vi "DmFET_Underway_Graphed.vi"() -> ()   [LabVIEW 2022 SP3]
uses:
  <vilib>/Utility/file.llb/Write Delimited Spreadsheet (string).vi
panel:
  out "TC_Controller":dbl
  out "BiasBatt- V":dbl
  out "BiasBatt+ V":dbl
  out "MainBatt V":dbl
  out "Ib":dbl
  out "Ik":dbl
  out "Vk_std":dbl
  out "Vk":dbl
  out "Vrse_std":dbl
  out "Vrse":dbl
  out "Vrse_std vs Time":waveform(dbl)(graph)
  out "Vrse vs Time":waveform(dbl)(graph)
  out "Loop #":i32
  in  "milliseconds to wait":u32=2000
  in  "stop":bool
  in  "file (use dialog)":path
  in  "DURA1 COM":refnum<visa-resource-name>="COM24"
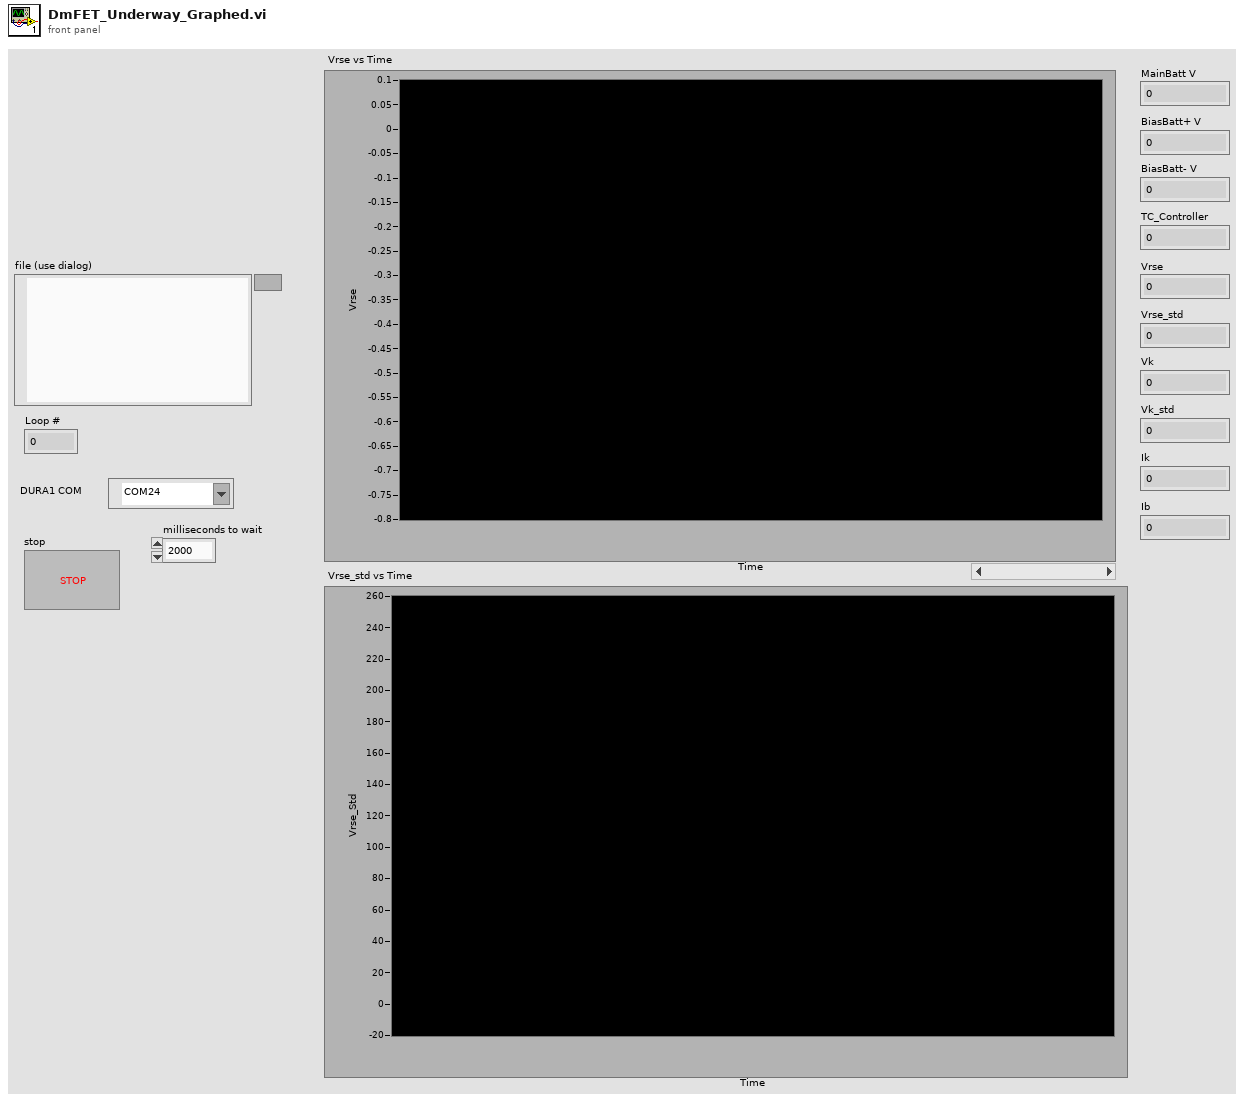
[diagram p1: front panel]
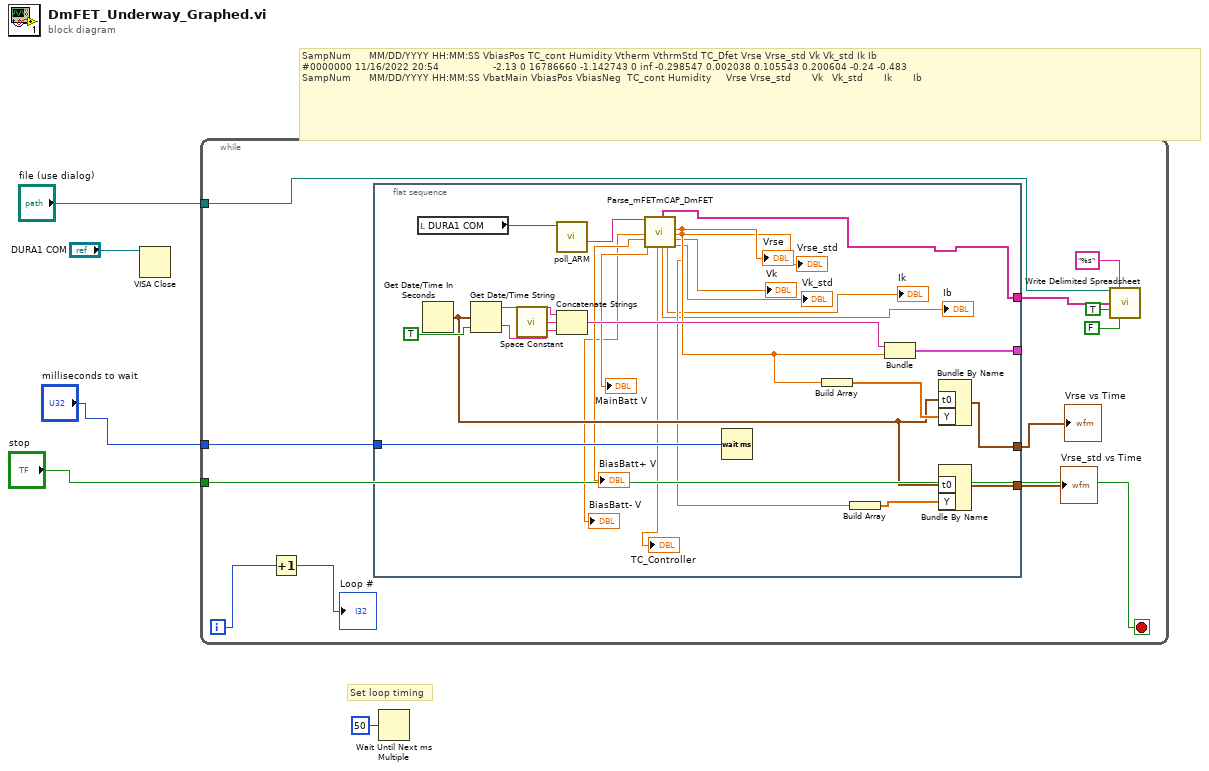
[diagram p0: block diagram]
diagram:
  # "Set loop timing"
  # "SampNum\t     MM/DD/YYYY HH:MM:SS\tVbiasPos\tTC_cont\tHumidity\tVtherm\tVthrmStd\tTC_Dfet\tVrse\tVrse_std\tVk\tVk_std\tIk\tIb\n#0000000\t11/16/2022 20:54                  -2.13\t0\t16786660\t-1.142743\t0\tinf\t-0.298547\t0.002038\t0.105543\t0.200604\t-0.24\t-0.483\nSampNum\t     MM/DD/YYYY HH:MM:SS\tVbatMain\tVbiasPos\tVbiasNeg\t TC_cont\tHumidity\t    Vrse\tVrse_std\t      Vk\t  Vk_std\t      Ik\t      Ib"
  n1 = VISA Close(VISA resource name="DURA1 COM") -> ()  [unwired: 1 in, 1 out]
  n2 = while {
    tunnel: "stop" -> [w16]
    tunnel: "file (use dialog)" -> [w9]
    tunnel: "milliseconds to wait" -> [w15]
    i -> [w14]
    stop <- w16 stop-if-true
    n3 = Increment(x=w14) -> (x+1=→"Loop #":i32)
    n4 = flat-sequence {
      tunnel: w15 -> [w40]
      tunnel: [w27] -> w8
      tunnel: [w38] -> _
      tunnel: [w31] -> w7
      tunnel: [w29] -> w6
      frame #0 {
        n5 = local read "DURA1 COM"() -> (w41:refnum<visa-resource-name>)
        n6 = Get Date/Time In Seconds() -> (seconds since 1Jan1904=w30:timestamp)
        n7 = Get Date/Time String(seconds (now)=w30, want seconds? (F)=TRUE) -> (date string=w36:string, time string=w35:string)  [unwired: 1 in]
        n8 = call <vilib>:"Space Constant.vi"() -> ("String"=w37:string)
        n9 = call "poll_ARM.vi"("ARM COM"=w41) -> ("ARM Reply"=w39:string)  [unwired: 10 in]
        n10 = Concatenate Strings(w36, w37, w35) -> (w33:string)
        n11 = call "Parse_mFETmCAP_DmFET.vi"("mFET_reply"=w39) -> ("BiasBatt- V"=→"BiasBatt- V":dbl, "BiasBatt+ V"=→"BiasBatt+ V":dbl, "MainBatt V"=→"MainBatt V":dbl, "TC_Controller"=→"TC_Controller":dbl, "Reply to save"=w27:string[], "Ib"=→"Ib":dbl, "Ik"=→"Ik":dbl, "Vrs_ext"=w26:dbl, "Vrs_ext std"=w25:dbl, "Vk"=→"Vk":dbl, "Vk std"=→"Vk_std":dbl)  [unwired: 6 in, 2 out]
        "Vrse" <- w26
        "Vrse_std" <- w25
        n12 = Wait (ms)(milliseconds to wait=w40) -> ()  [unwired: 1 out]
        n13 = Build Array(w26) -> (w32:dbl[])
        n14 = Build Array(w25) -> (w28:dbl[])
        n15 = Bundle(w33, "Vrs_ext"=w26) -> (w38:cluster{string, "Vrs_ext":dbl})  [unwired: 1 in]
        n16 = Bundle By Name("t0"=w30, "Y"=w32) -> (w31:waveform(dbl))  [unwired: 1 in]
        n17 = Bundle By Name("t0"=w30, "Y"=w28) -> (w29:waveform(dbl))  [unwired: 1 in]
      }
    }
    n18 = call-poly <vilib>:"Write Delimited Spreadsheet.vi"("file path (dialog if empty)"=w9, "format (%s)"="%s" ("format (%.3f)"), "1D data"=w8, "append to file? (new file:F)"=TRUE, "transpose? (no:F)"=FALSE) -> ()  [unwired: 9 in, 2 out]
    "Vrse vs Time" <- w7
    "Vrse_std vs Time" <- w6
  }
  n19 = Wait Until Next ms Multiple(millisecond multiple=u32 50) -> ()  [unwired: 1 out]
